vi "UI Pre-Build Action.vi"(6 "Top Level/Always Included VIs":path[](array[path]), 7 "Main Destination Path":path, 9 "Target Name":string, 10 "Build Specification Name":string, 11 "Project Path":path) -> (0 "error out":errorcluster)   [LabVIEW 2021, in "CIF Build Actions.lvlib"]
uses:
  CIF Build Actions.lvlib
  <vilib>/AppBuilder/AB_API/common/AB_API Build Object Selector.ctl
  <vilib>/AppBuilder/AB_API/PPL/NI_AB_API_PPL.lvclass
  CIFCore/Common/Typedef/Errors.ctl
  <vilib>/CIF Foundation/CIF Utilities/Errors/Append Error Location.vi
  <vilib>/AppBuilder/AB_API/Build/NI_AB_API_Build.lvclass
  CIFCore/Common/CIFCoreCommon.lvlib
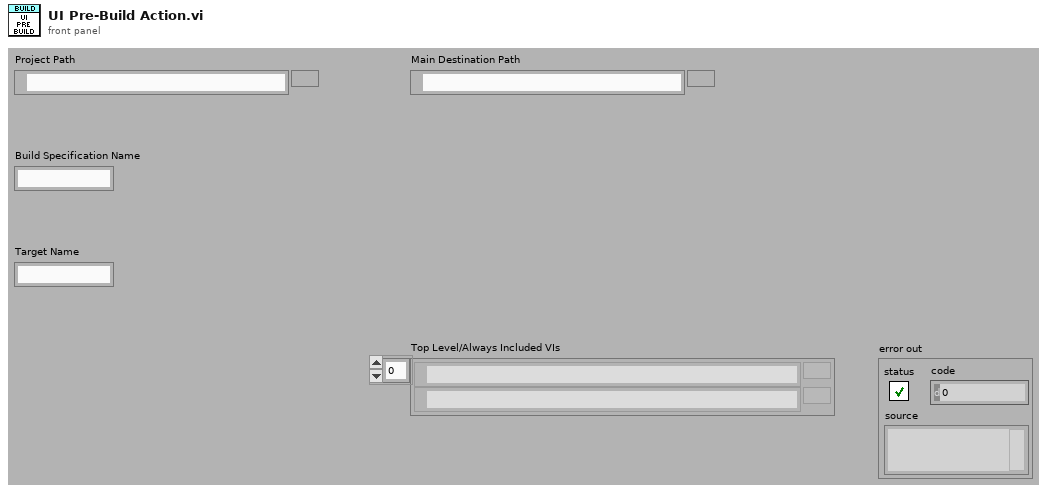
[diagram p1: front panel]
types:
  T1 = cluster{"Major":u16, "Minor":u16, "Fix":u16, "Build":u16}
  T2 = typedef "AB_API Build Object Selector.ctl" = enum16{"Source Distribution", "Deployable Source Distribution", "DLL", "EXE", "Packed Library", "Deployable Packed Library", "RT EXE", ".NET Interop Assembly"}
  T3 = typedef "CIFCoreCommon.lvlib/Errors.ctl" = enum16{"Invalid Clock ID", "Long Sleep", "gRPC Server Not Found", "Config Parse", "Timestamp Wrap", "Delayed Execution", "Duplicate Channel", "Missing Channel", "Incorrect Type", "Flatten Error", "Unflatten Data", "Unique Name", "Plugin Not Found", "Plugin Type Not Found", "Plugin Version Not Found", "Manager Not Found", "Numerical Issue", "Time Jump", "Clock ID Match", "Channel Length", "Plugin Connection", "gRPC Server Connection", "PPL Name Match", "Build", "Config Log Parse"}
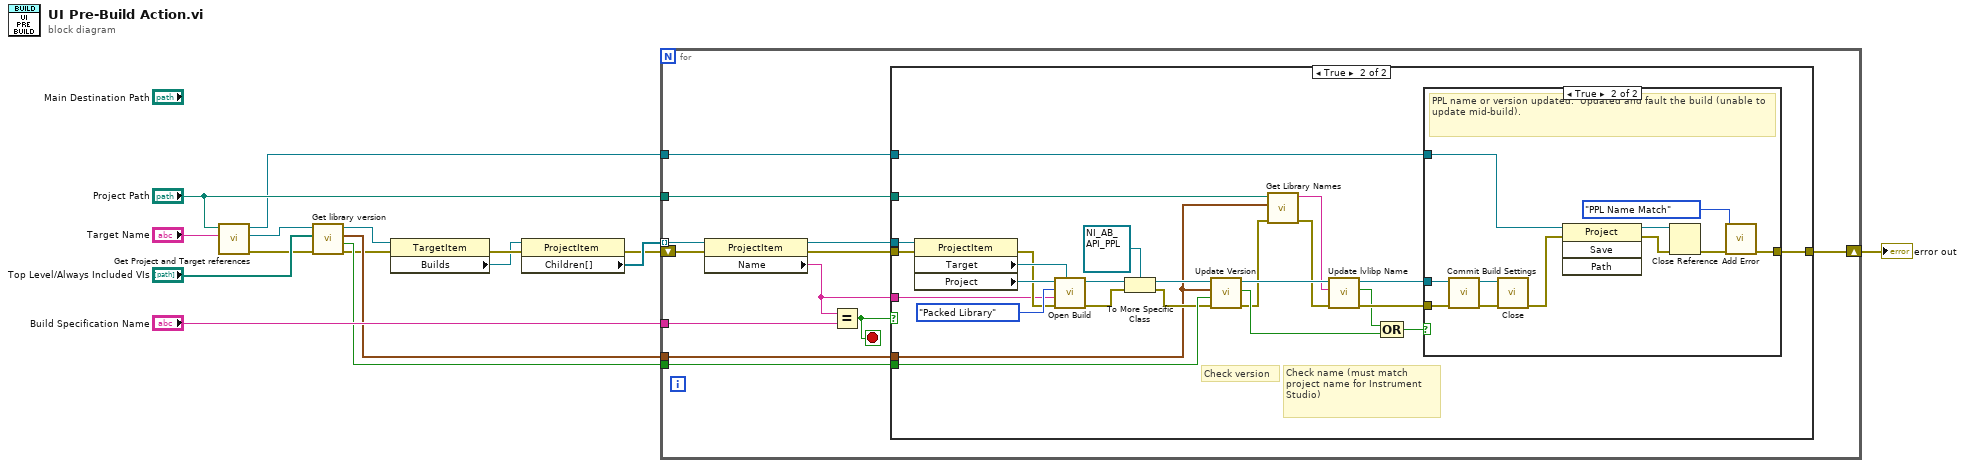
[diagram p0: block diagram]
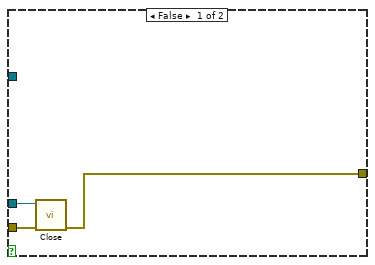
[diagram p3: hidden frame]
diagram:
  n1 = call "Get Project and Target references.vi"("Target Name"="Target Name", "Project Path"="Project Path") -> ("error out"=w5:errorcluster, "Target refnum"=w7:refnum<vi>, "Project refnum"=w1:refnum<vi>)  [unwired: 7 in]
  n2 = call "Get library version.vi"("error in (no error)"=w5, "Top Level/Always Included VIs"="Top Level/Always Included VIs", "Target reference in"=w7) -> ("error out"=w2:errorcluster, "Library Found"=w8:bool, "Version"=w9:T1, "Target reference out"=w6:refnum<vi>)  [unwired: 4 in, 1 out]
  n3 = property class="TargetItem"(reference=w6, error in=w2) -> (error out=w15:errorcluster, "Builds"=w14:refnum<vi>)  [unwired: 1 out]
  n4 = property class="ProjectItem"(reference=w14, error in=w15) -> (error out=w4:errorcluster, "Children[]"=w16:refnum<vi>[])  [unwired: 1 out]
  n5 = for {
    tunnel: w16 -> [w27] mode=indexing
    tunnel: w9 -> [w28]
    tunnel: w8 -> [w21]
    shift-right: [w23] -> w12
    shift-left: w4 -> [w24]
    tunnel: w1 -> [w19]
    tunnel: "Build Specification Name" -> [w18]
    tunnel: "Project Path" -> [w17]
    stop <- w20 stop-if-true
    n6 = property class="ProjectItem"(reference=w27, error in=w24) -> (reference out=w26:refnum<vi>, error out=w25:errorcluster, "Name"=w22:string)
    n7 = Equal?(x=w22, y=w18) -> (x = y?=w20:bool)
    n8 = case shown="True" w20 {
      tunnel: w28 -> [_ w33]
      tunnel: w26 -> [_ w48]
      tunnel: w25 -> [w29 w47]
      tunnel: [w29 w46] -> w23
      tunnel: w22 -> [_ w44]
      tunnel: w21 -> [_ w45]
      tunnel: w19 -> [_ w43]
      tunnel: w17 -> [_ w34]
      frame False {
      }
      frame True {
        # "Check name (must match project name for Instrument Studio)"
        # "Check version"
        n9 = property class="ProjectItem"(reference=w48, error in=w47) -> (error out=w49:errorcluster, "Target"=w55:refnum<vi>, "Project"=w54:refnum<vi>)  [unwired: 1 out]
        n10 = call <vilib>:"Open Build.vi"("TargetItem Refnum"=w55, "error in (no error)"=w49, "Build specification name"=w44, "Build object selector"=AB_API_Build_Object_Selector."Packed Library", "Project Refnum"=w54) -> ("error out"=w50:errorcluster, "NI_AB_API_Build out"=w52:refnum<class "NI_AB_API_Build.lvclass">)  [unwired: 5 in]
        n11 = To More Specific Class(target class=refnum<class "NI_AB_API_PPL.lvclass"> refnum ("PPL out"), reference=w52, error in=w50) -> (specific class reference=w42:refnum<class "NI_AB_API_PPL.lvclass">, error out=w41:errorcluster)
        n12 = call "Update Version.vi"("error in (no error)"=w41, "Valid"=w45, "Library Version"=w33, "NI_AB_API_PPL in"=w42) -> ("error out"=w32:errorcluster, "Updated"=w36:bool, "NI_AB_API_PPL out"=w40:refnum<class "NI_AB_API_PPL.lvclass">)  [unwired: 5 in]
        n13 = call "Get Library Names.vi"("error in (no error)"=w32, "Version"=w33, "Project Path"=w34) -> ("error out"=w30:errorcluster, "Library"=w31:string)  [unwired: 5 in, 2 out]
        n14 = call "Update lvlibp Name.vi"("error in (no error)"=w30, "lvlibp name"=w31, "NI_AB_API_PPL in"=w40) -> ("error out"=w39:errorcluster, "Updated"=w37:bool, "NI_AB_API_PPL out"=w38:refnum<class "NI_AB_API_PPL.lvclass">)  [unwired: 6 in]
        n15 = Compound Arithmetic op=OR(w37, w36) -> (w35:bool)
        n16 = case shown="True" w35 {
          tunnel: [w58 w63] -> w46
          tunnel: w43 -> [_ w59]
          tunnel: w39 -> [w56 w61]
          tunnel: w38 -> [w57 w60]
          frame False {
            n17 = call-dynamic "Close.vi"("error in (no error)"=w56, "DLL in"=w57) -> ("error out"=w58:errorcluster)  [unwired: 9 in]
          }
          frame True {
            # "PPL name or version updated.  Updated and fault the build (unable to update mid-build)."
            n18 = call-dynamic "Commit Build Settings.vi"("error in (no error)"=w61, "PPL in"=w60) -> ("error out"=w68:errorcluster, "PPL out"=w69:refnum<class "NI_AB_API_PPL.lvclass">)  [unwired: 8 in]
            n19 = call-dynamic "Close.vi"("error in (no error)"=w68, "DLL in"=w69) -> ("error out"=w65:errorcluster)  [unwired: 9 in]
            n20 = invoke class="Project" method="Save"(reference=w59, error in=w65) -> (reference out=w66:refnum<vi>, error out=w67:errorcluster)  [unwired: 2 in, 2 out]
            n21 = Close Reference(reference=w66, error in (no error)=w67) -> (error out=w64:errorcluster)
            n22 = call "Add Error.vi"("error in (no error)"=w64, "Error"=Errors."PPL Name Match") -> ("error out"=w63:errorcluster)  [unwired: 9 in]
          }
        }
      }
    }
  }
  "error out" <- w12
